vi "Vision Processing.vi"(4 "error in (no error)":errorcluster, 6 "CameraDevRef":T1) -> ()   [LabVIEW 2011]
uses:
  <vilib>/Rock Robotics/WPI/Camera/WPI_CameraDevRef.ctl
  Robot Global Data.vi
  <vilib>/vision/NI_Vision_Development_Module.lvlib
panel:
  in  "Y AbsolVal Difference":dbl=0.25
  in  "Default Shooter Speed Dump":dbl=0.42
  in  "Default Shooter Speed Shoot":dbl=1.0
  in  "Scale":dbl=0.85
  in  "Minimum Power":dbl=0.22
  out "Aspect Ratio":dbl[](array[numeric])
  out "Offset":dbl
  out "Raw Turret":dbl
  out "Target X Coord":dbl
  out "Target Distance":dbl
  out "Distance Array":dbl[](array[numeric])
  in  "Dead Band":dbl=0.09
  out "Number of Rectangles Visible":dbl
  out "Y Position Array":dbl[](array[numeric])
  out "X Position Array":dbl[](array[numeric])
  in  "View":bool
  out "Target Info":T2(array[cluster])
  in  "Area Size Limit":i32=444
  in  "Particle Count Limit":i32=8
  in  "Score Limits":T3={"Rect Coverage"=76.0, "Aspect Ratio"=40.0, "X Edge Strength"=40.0, "Y Edge Strength"=60.0}
  in  "Processing":enum32{"Color", "Intensity", "Intensity Open"}(tab)=enum."Intensity"
  in  "Luminance":i32=255
  in  "Saturation":i32=255
  in  "Hue":i32(knob)=65 scale=0.0..255.0
  in  "Margins":cluster{"Hue":i32, "Sat":i32, "Lum":i32}={"Hue"=20, "Sat"=27, "Lum"=30} {"Sat" scale=0.0..40.0; "Lum" scale=0.0..40.0; "Hue" scale=0.0..40.0}
  in  "Range":cluster{"Lower value":sgl, "Upper value":sgl}={"Lower value"=151.52174, "Upper value"=255.0} {"Lower value" scale=0.0..255.0; "Upper value" scale=0.0..255.0}
  in  "Range":cluster{"Lower value":sgl, "Upper value":sgl}={"Lower value"=123.804344, "Upper value"=255.0} {"Lower value" scale=0.0..255.0; "Upper value" scale=0.0..255.0}
  in  "View":bool
  out "Processed Image":T4(plugin-control)
  out "Original Image":T4(plugin-control)
  # "Instructions:\nProcessing the reflective tape that is illuminated by a ring light can be based\non color or light intensity.\nParticles within the image are scored by rectangle coverage, aspect ratio, and\nfor being hollow with a bold edge. A particle is considered a target if all scores\nare above the score limits. Particles can be annotated -- surrounded by\na rectangle and scores drawn to the left .\nTo control the number of particles being scored, use the count limit and the size\nlimit."
  # "(in)"
  # "To debug, Enable using the View button.\nFor color processing, you can click in the image to select the color for processing."
  # "Enable by clicking the View button.\nGreen scores are above the limit, orange are below. Inner/outer rect\nindicates all passed."
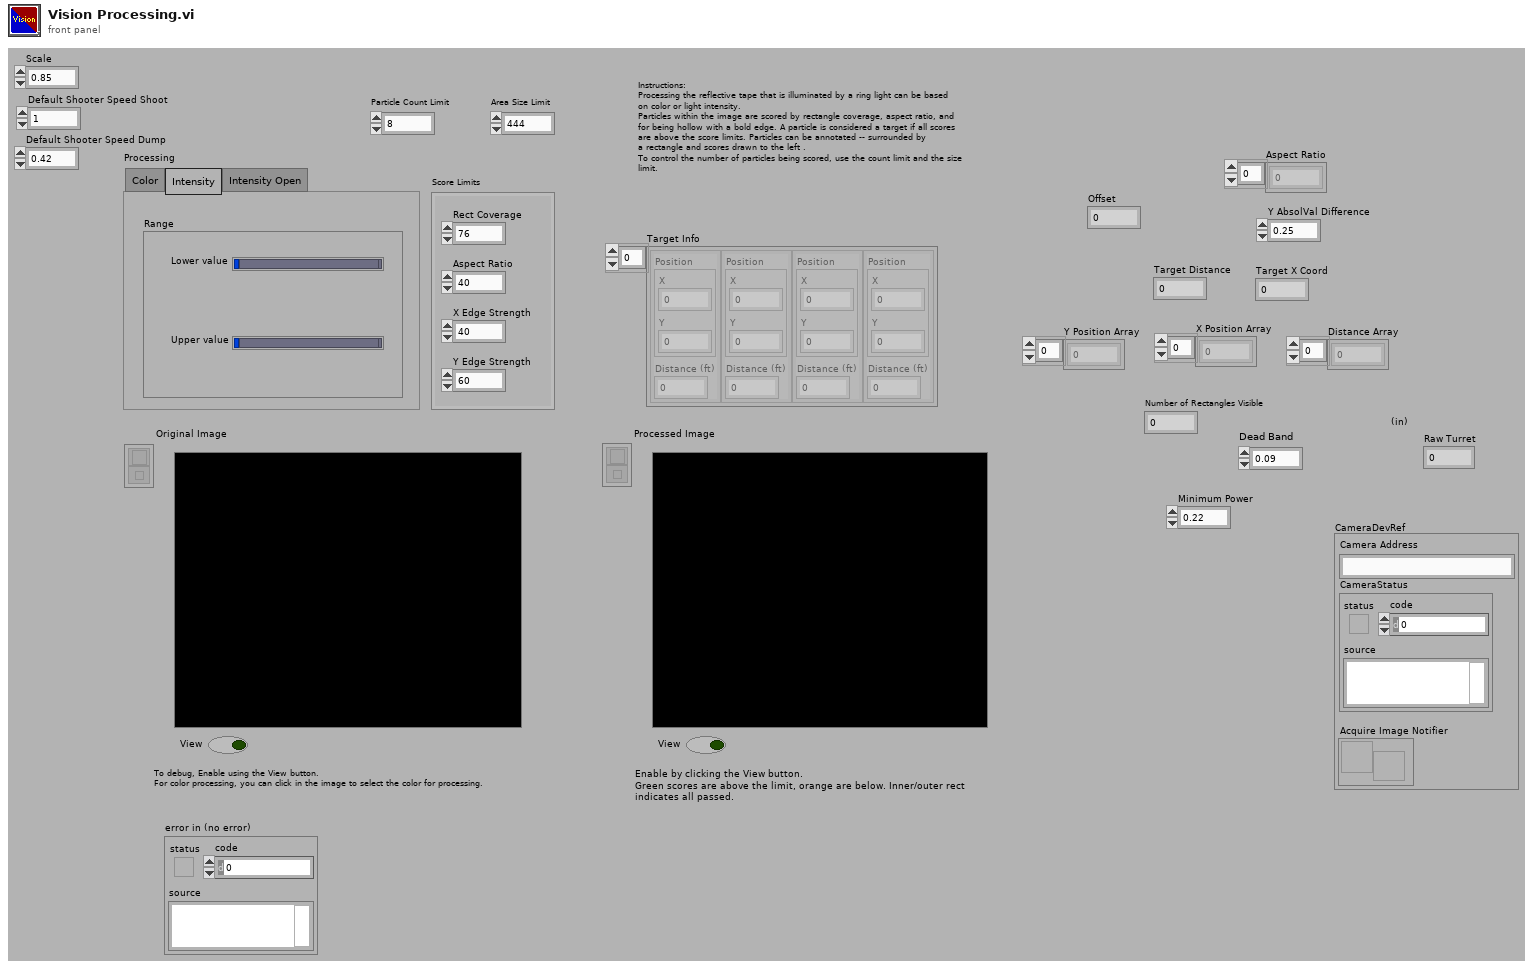
[diagram p1: front panel]
types:
  T1 = typedef "WPI_CameraDevRef.ctl" = cluster{"Camera Address":string, "CameraStatus":errorcluster, "Acquire Image Notifier":refnum<notifier>}
  T2 = cluster{"Position":cluster{"X":dbl, "Y":dbl}, "Distance (ft)":dbl}[]
  T3 = cluster{"Rect Coverage":dbl, "Aspect Ratio":dbl, "X Edge Strength":dbl, "Y Edge Strength":dbl}
  T4 = typedef "IMAQ Image.ctl" = refnum<image>
  T5 = typedef "Image Type" = u32
  T6 = enum32{"AutoM", "Close", "Dilate", "Erode", "Gradient", "Gradient out", "Gradient in", "Hit miss", "Open", "PClose", "POpen", "Thick", "Thin"}
  T7 = typedef "WPI_CameraImageSize.ctl" = enum16{"640x480", "320x240", "160x120"}
  T8 = cluster{"fps":i32, "compression":i32, "Image Size":T7}
  T9 = cluster{cluster{"Left":dbl, "Top":dbl, "Right":dbl, "Bottom":dbl}, dbl[]}[]
  T10 = cluster{"Left":dbl, "Top":dbl, "Right":dbl, "Bottom":dbl}
  T11 = cluster{"Target Center (-1 to 1)":cluster{"X":dbl, "Y":dbl}, "Distance (ft)":dbl}
  T12 = cluster{"Target Center (-1 to 1)":cluster{"X":dbl, "Y":dbl}, "Distance (ft)":dbl}[]
  T13 = typedef "WPI_JoystickDevRef.ctl" = cluster{"Device":T14}
  T14 = typedef "WPI_JoystickDeviceEnum.ctl" = enum16{"USB 1", "USB 2", "USB 3", "USB 4", "Kinect 1", "Kinect 2"}
  T15 = typedef "WPI_JoystickButtonState.ctl" = cluster{"Button 1":bool, "Button 2":bool, "Button 3":bool, "Button 4":bool, "Button 5":bool, "Button 6":bool, "Button 7":bool, "Button 8":bool, "Button 9":bool, "Button 10":bool, "Button 11":bool, "Button 12":bool}
  T16 = cluster{"axis 1 (x)":dbl, "axis 2 (y)":dbl, "axis 3 (throttle)":dbl, "axis 4":dbl, "axis 5":dbl, "axis 6":dbl}
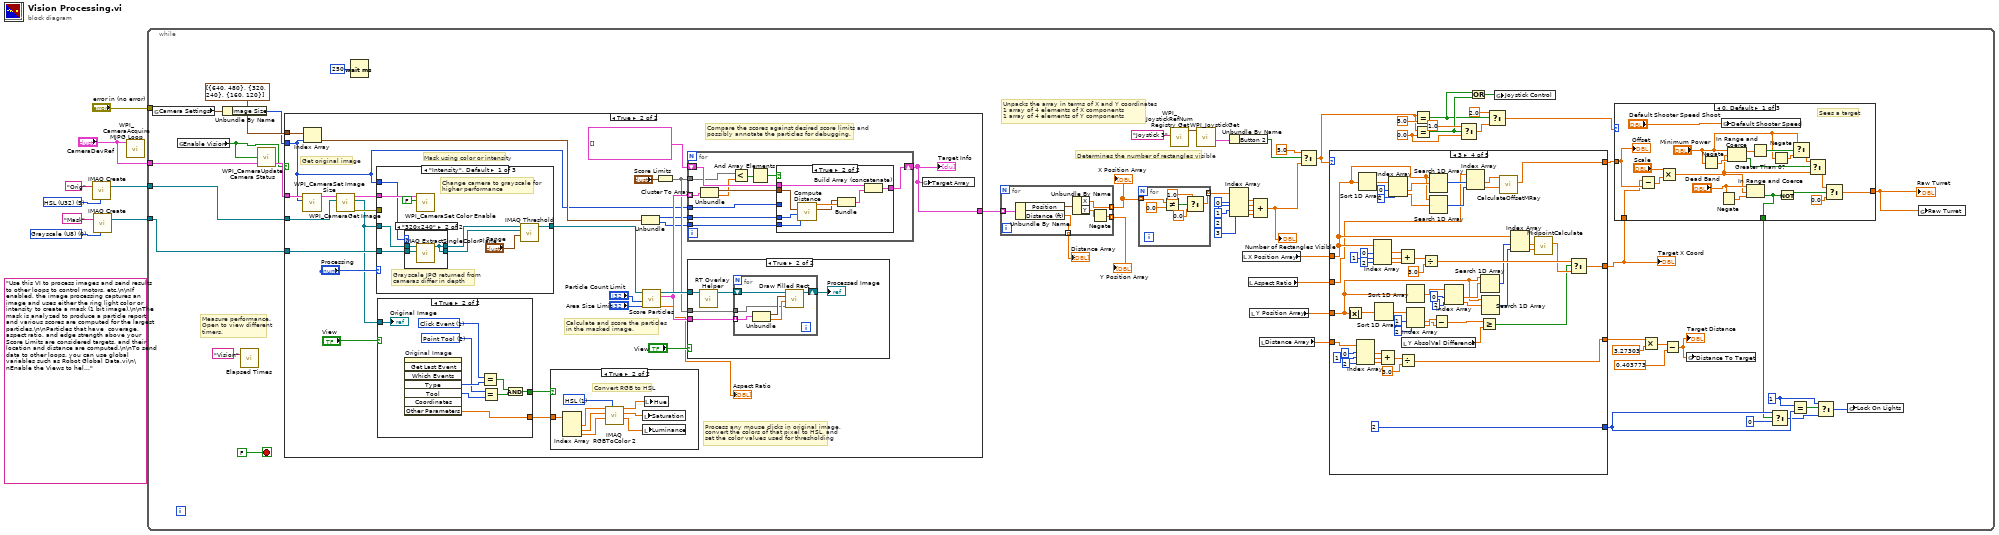
[diagram p0: block diagram]
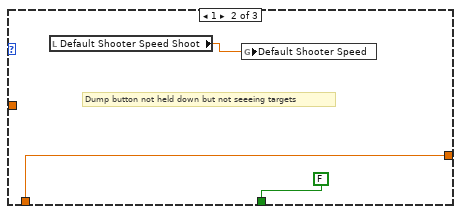
[diagram p2: hidden frame]
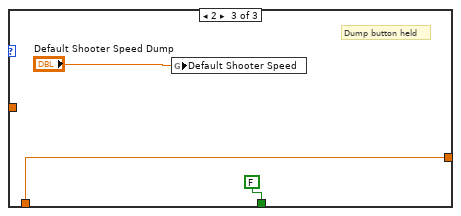
[diagram p3: hidden frame]
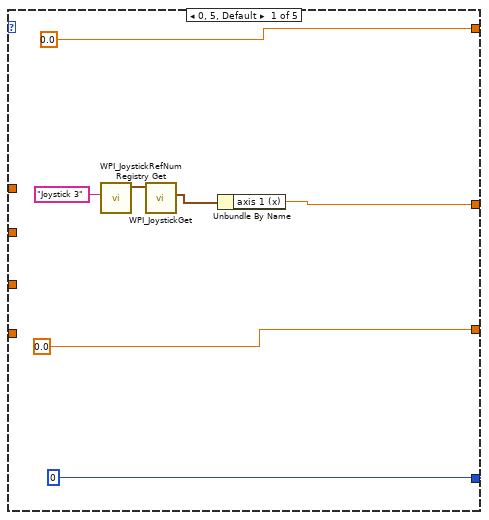
[diagram p4: hidden frame]
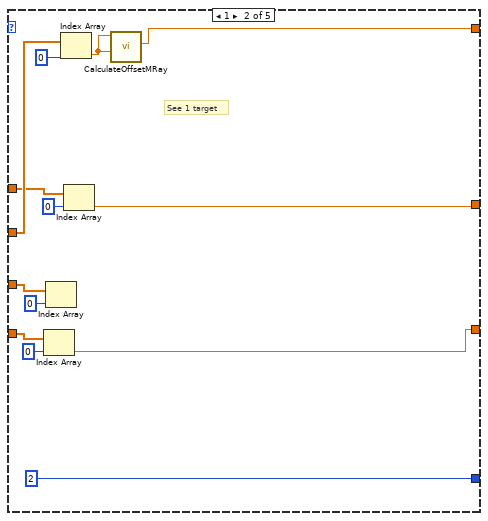
[diagram p5: hidden frame]
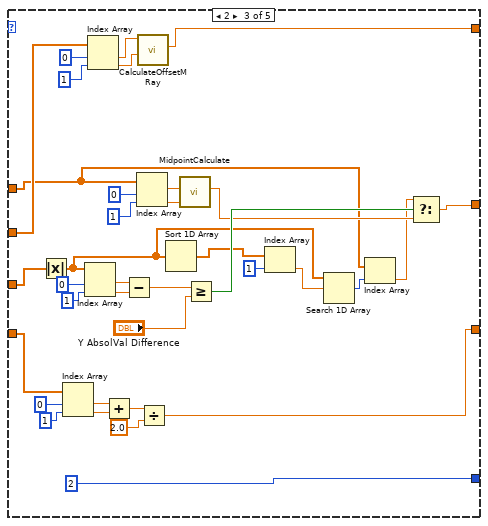
[diagram p6: hidden frame]
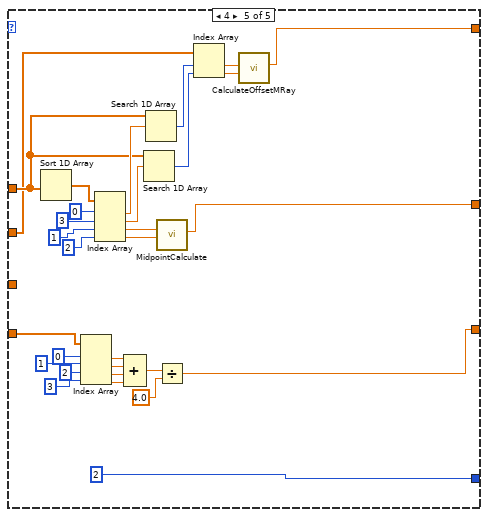
[diagram p7: hidden frame]
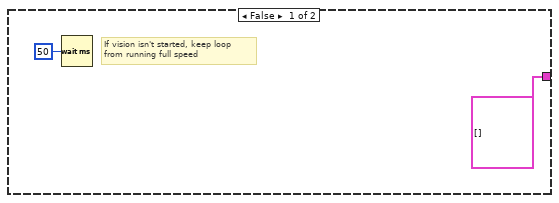
[diagram p8: hidden frame]
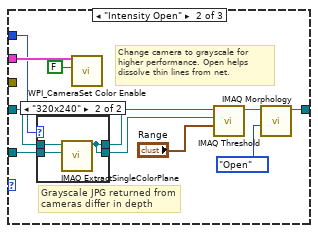
[diagram p11: hidden frame]
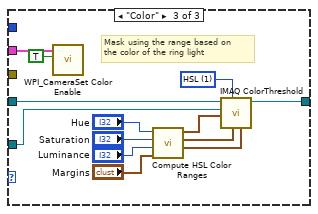
[diagram p13: hidden frame]
diagram:
  w3 = T5 0 items=["Grayscale (U8)", "Grayscale (I16)", "Grayscale (SGL)", "Complex (CSG)", "RGB (U32)", "HSL (U32)", "RGB (U64)", "Grayscale (U16)"] ("Image Type")
  (unwired) "Use this VI to process images and send results to other loops to control motors, etc.\n\nIf enabled, the image processing captures an image and uses either the ring light color or intensity to create a mask (1 bit image).\n\nThe mask is analyzed to produce a particle report and various scores are computed for the largest particles.\n\nParticles that have  coverage, aspect ratio, and edge strength above your Score Limits are considered targets, and their location and distance are computed.\n\nTo send data to other loops, you can use global variables such as Robot Global Data.vi\n\nEnable the Views to help debug color settings. Disable the View to speed up processing."
  w7 = T5 5 items=["Grayscale (U8)", "Grayscale (I16)", "Grayscale (SGL)", "Complex (CSG)", "RGB (U32)", "HSL (U32)", "RGB (U64)", "Grayscale (U16)"] ("Image Type")
  n1 = call "IMAQ Create"("Image Name"="Orig", "Image Type"=w7) -> ("New Image"=w6:T4)  [unwired: 2 in, 2 out]
  n2 = call "IMAQ Create"("Image Name"="Mask", "Image Type"=w3) -> ("New Image"=w1:T4)  [unwired: 2 in, 2 out]
  n3 = call <vilib>:"WPI_CameraAcquire MJPG Loop.vi"("CameraDevRef"="CameraDevRef") -> ()  [unwired: 11 in]
  n4 = while {
    tunnel: w6 -> [w66]
    tunnel: "CameraDevRef" -> [w65]
    tunnel: "error in (no error)" -> [_]
    tunnel: w1 -> [w61]
    stop <- FALSE stop-if-true
    w14 = 0.0 ("y")
    w31 = 1 ("y")
    # "Determines the number of rectangles visible"
    # "Unpacks the array in terms of X and Y coordinates\n1 array of 4 elements of X components\n1 array of 4 elements of Y components"
    # "Measure performance.\nOpen to view different\ntimers."
    n5 = global read "Robot Global Data.vi" "Camera Settings"() -> (w59:T8)
    n6 = global read "Robot Global Data.vi" "Enable Vision"() -> (w63:bool)
    n7 = Unbundle By Name(w59) -> ("Image Size"=w58:T7)
    n8 = call "Elapsed Times.vi"("Call Name"="Vision") -> ()  [unwired: 2 in, 1 out]
    n9 = call <vilib>:"WPI_CameraUpdate Camera Status.vi"("CameraDevRef In"=w65, "Enable Vision"=w63) -> ("CameraDevRef Out"=w64:T1)  [unwired: 3 in]
    n10 = case shown="True" w63 {
      tunnel: w66 -> [_ w264]
      tunnel: w64 -> [_ w260]
      tunnel: w61 -> [_ w251]
      tunnel: cluster{i32, i32}[] [{640, 480}, {320, 240}, {160, 120}] -> [_ w255]
      tunnel: w58 -> [_ w248]
      tunnel: [T2 [] w249] -> w57
      frame False {
        # "If vision isn't started, keep loop\nfrom running full speed"
        n11 = Wait (ms)(milliseconds to wait=u32 50) -> ()  [unwired: 1 out]
      }
      frame True {
        # "Compare the scores against desired score limits and\npossibly annotate the particles for debugging."
        # "Process any mouse clicks in original image,\nconvert the colors of that pixel to HSL, and\nset the color values used for thresholding"
        # "Calculate and score the particles\nin the masked image."
        # "Mask using color or intensity"
        # "Get original image"
        n12 = call <vilib>:"WPI_CameraSet Image Size.vi"("Image Size"=w248, "CameraDevRef"=w260) -> ("CameraDevRef Out"=w261:T1)  [unwired: 8 in, 1 out]
        n13 = Index Array(array=w255, index=w248) -> (element=w252:cluster{i32, i32})
        n14 = call <vilib>:"WPI_CameraGet Image.vi"("Image"=w264, "CameraDevRef"=w261) -> ("error out"=w262:errorcluster, "Image Out"=w250:T4, "CameraDevRef Out"=w263:T1)  [unwired: 7 in]
        n15 = case shown="\"Intensity\", Default" "Processing" {
          tunnel: w250 -> [w286 w298 w324]
          tunnel: [w289 w303 w323] -> w258
          tunnel: w263 -> [w287 w301 w314]
          tunnel: w262 -> [_ _ _]
          tunnel: w251 -> [w285 w299 w312]
          tunnel: w248 -> [w284 w300 _]
          frame "Intensity", Default {
            # "Grayscale JPG returned from\ncameras differ in depth"
            # "Change camera to grayscale for\nhigher performance"
            n16 = case shown="\"320x240\"" w284 {
              tunnel: w286 -> [w292 w295]
              tunnel: w285 -> [w291 w294]
              tunnel: [w292 w293] -> w283
              tunnel: [w291 w293] -> w282
              frame "640x480", Default {
              }
              frame "320x240" {
                n17 = call "IMAQ ExtractSingleColorPlane"("Image Dst"=w294, "Image Src"=w295) -> ("Image Dst Out"=w293:T4)  [unwired: 8 in, 1 out]
              }
            }
            n18 = call <vilib>:"WPI_CameraSet Color Enable.vi"("Color Enabled"=FALSE, "CameraDevRef"=w287) -> ()  [unwired: 8 in, 2 out]
            n19 = call "IMAQ Threshold"("Range"="Range", "Image Dst"=w282, "Image Src"=w283) -> ("Image Dst Out"=w289:T4)  [unwired: 3 in, 5 out]
          }
          frame "Intensity Open" {
            # "Grayscale JPG returned from\ncameras differ in depth"
            # "Change camera to grayscale for\nhigher performance. Open helps\ndissolve thin lines from net."
            n20 = case shown="\"320x240\"" w300 {
              tunnel: w298 -> [w308 w311]
              tunnel: w299 -> [w307 w310]
              tunnel: [w308 w309] -> w297
              tunnel: [w307 w309] -> w296
              frame "640x480", Default {
              }
              frame "320x240" {
                n21 = call "IMAQ ExtractSingleColorPlane"("Image Dst"=w310, "Image Src"=w311) -> ("Image Dst Out"=w309:T4)  [unwired: 8 in, 1 out]
              }
            }
            n22 = call <vilib>:"WPI_CameraSet Color Enable.vi"("Color Enabled"=FALSE, "CameraDevRef"=w301) -> ()  [unwired: 8 in, 2 out]
            n23 = call "IMAQ Threshold"("Range"="Range", "Image Dst"=w296, "Image Src"=w297) -> ("Image Dst Out"=w304:T4)  [unwired: 3 in, 5 out]
            n24 = call "IMAQ Morphology"("Operation"=T6."Open", "Image Src"=w304) -> ("Image Dst Out"=w303:T4)  [unwired: 8 in, 1 out]
          }
          frame "Color" {
            w322 = u16 1 items=["RGB", "HSL", "HSV", "HSI"] ("Color Mode")
            # "Mask using the range based on\nthe color of the ring light"
            n25 = call <vilib>:"WPI_CameraSet Color Enable.vi"("Color Enabled"=TRUE, "CameraDevRef"=w314) -> ()  [unwired: 8 in, 2 out]
            n26 = call "Compute HSL Color Ranges.vi"("Margins"="Margins", "Luminance"="Luminance", "Saturation"="Saturation", "Hue"="Hue") -> ("Lum Range"=w319:cluster{i32, i32}, "Sat Range"=w320:cluster{i32, i32}, "Hue Range"=w321:cluster{i32, i32})  [unwired: 5 in]
            n27 = call "IMAQ ColorThreshold"("Blue or Luma or Val or Inten Range"=w319, "Green or Sat Range"=w320, "Color Mode"=w322, "Red or Hue Range"=w321, "Image Dst"=w312, "Image Src"=w324) -> ("Image Dst Out"=w323:T4)  [unwired: 4 in, 1 out]
          }
        }
        n28 = case shown="True" "View" {
          tunnel: w250 -> [_ w344]
          tunnel: [_ w339] -> w257
          tunnel: [_ w336] -> w256
          frame False {
          }
          frame True {
            w337 = 2 items=["None", "Selection Tool", "Point Tool", "Line Tool", "Rectangle Tool", "Oval Tool", "Polygon Tool", "ClosedFreehandTool", "Annulus Tool", "Rotated Rectangle Tool", "Zoom Tool", "Pan Tool", "Polyline Tool", "Freehand Tool"] ("Tool")
            w338 = 1 items=["No Event"=0, "Click Event"=1, "Draw Event"=2, "Size Event"=4, "Scroll Event"=5, "Double Click Event"=8] ("Type")
            n29 = invoke on="Original Image" class="ImageControl" method="Get Last Event"() -> ("Type"=w340:i32, "Tool"=w343:i32, "Other Parameters"=w336:sgl[])  [unwired: 8 in, 5 out]
            n30 = Equal?(x=w338, y=w340) -> (x = y?=w341:bool)
            n31 = Equal?(x=w337, y=w343) -> (x = y?=w342:bool)
            n32 = And(x=w341, y=w342) -> (x .and. y?=w339:bool)
            "Original Image" <- w344
          }
        }
        n33 = case shown="True" w257 {
          tunnel: w256 -> [_ w281]
          frame False {
          }
          frame True {
            w280 = u16 1 items=["RGB", "HSL", "HSV", "HSI", "CIE L*a*b*", "CIE XYZ"] ("Color Mode")
            # "Convert RGB to HSL"
            n34 = Index Array(array=w281) -> (element #1=w279:sgl, element #2=w277:sgl, element #3=w275:sgl)  [unwired: 3 in]
            n35 = call "IMAQ RGBToColor 2"("Color Mode"=w280, "Blue value"=w275, "Green value"=w277, "Red value"=w279) -> ("Blue or Luma or Val or Inten or Z or b*value"=w274:dbl, "Green or Sat or Y or a* value"=w276:dbl, "Red or Hue or X or L* value"=w278:dbl)  [unwired: 4 in, 1 out]
            n36 = local write "Saturation"(w276) -> ()
            n37 = local write "Luminance"(w274) -> ()
            n38 = local write "Hue"(w278) -> ()
          }
        }
        n39 = Unbundle(w252) -> (w254:i32, w253:i32)
        n40 = call "Score Particles.vi"("Area Size Limit"="Area Size Limit", "Particle Count Limit"="Particle Count Limit", "Image Refnum in"=w258) -> ("Aspect Ratio"=→"Aspect Ratio":dbl[], "Scored Particle Info"=w269:T9, "Image Refnum out"=w272:T4)  [unwired: 6 in]
        n41 = Cluster To Array(cluster="Score Limits") -> (array=w267:dbl[])
        n42 = for {
          shift-right: [w354] -> w249
          shift-left: T2 [] -> [w355]
          tunnel: w254 -> [w353]
          tunnel: w269 -> [w351] mode=indexing
          tunnel: w267 -> [w346]
          tunnel: w248 -> [w350]
          tunnel: w253 -> [w345]
          n43 = Unbundle(w351) -> (w352:T10, w347:dbl[])
          n44 = Less?(x=w346, y=w347) -> (x < y?=w349:bool[])
          n45 = And Array Elements(Boolean array=w349) -> (logical AND=w348:bool)
          n46 = case shown="True" w348 {
            tunnel: w355 -> [w356 w364]
            tunnel: [w356 w363] -> w354
            tunnel: w352 -> [_ w359]
            tunnel: w353 -> [_ w361]
            tunnel: w350 -> [_ _]
            tunnel: w345 -> [_ w358]
            frame False {
            }
            frame True {
              n47 = call "Compute Distance.vi"("Y Image Resolution"=w358, "X Image Resolution"=w361, "Bounding Box"=w359) -> ("Target Center (-1 to 1)"=w357:cluster{"X":dbl, "Y":dbl}, "Distance (ft)"=w360:dbl)  [unwired: 7 in]
              n48 = Bundle("Target Center (-1 to 1)"=w357, "Distance (ft)"=w360) -> (w362:T11)  [unwired: 1 in]
              n49 = Build Array (concatenate)(w364, w362) -> (w363:T12)
            }
          }
        }
        "Target Info" <- w249
        n50 = case shown="True" "View" {
          tunnel: w272 -> [_ w326]
          tunnel: w269 -> [_ w328]
          tunnel: w267 -> [_ w327]
          frame False {
          }
          frame True {
            n51 = call "RT Overlay Helper.vi"("Refnum in"=w326) -> ("Refnum out"=w329:T4)  [unwired: 10 in]
            n52 = for {
              shift-right: [w334] -> w325
              shift-left: w329 -> [w335]
              tunnel: w328 -> [w331] mode=indexing
              tunnel: w327 -> [w330]
              n53 = Unbundle(w331) -> (w332:T10, w333:dbl[])
              n54 = call "Draw Filled Rect.vi"("Limits"=w330, "Scores"=w333, "Bounding Box"=w332, "image in"=w335) -> ("image out"=w334:T4)  [unwired: 7 in]
            }
            "Processed Image" <- w325
          }
        }
        n55 = global write "Robot Global Data.vi" "Target Array"(w249) -> ()
      }
    }
    n56 = Wait (ms)(milliseconds to wait=u32 250) -> ()  [unwired: 1 out]
    n57 = for {
      tunnel: [w242] -> w37 mode=indexing
      tunnel: [w243] -> w47 mode=indexing
      tunnel: w57 -> [w240] mode=indexing
      tunnel: [w239] -> w49 mode=indexing
      n58 = Unbundle By Name(w240) -> ("Position"=w244:cluster{"X":dbl, "Y":dbl}, "Distance (ft)"=w239:dbl)
      n59 = Unbundle By Name(w244) -> ("X"=w243:dbl, "Y"=w241:dbl)
      n60 = Negate(x=w241) -> (-x=w242:dbl)
    }
    "X Position Array" <- w47
    "Y Position Array" <- w37
    "Distance Array" <- w49
    n61 = for {
      tunnel: w47 -> [w98] mode=indexing
      tunnel: [w94] -> w46 mode=indexing
      n62 = Not Equal?(x=w98, y=0.0) -> (x != y?=w97:bool)
      n63 = Select(t=1.0, s=w97, f=0.0) -> (s? t:f=w94:dbl)
    }
    n64 = call <vilib>:"WPI_JoystickRefNum Registry Get.vi"("refnum name"="Joystick 3") -> ("JoystickDevRef"=w36:T13)  [unwired: 9 in, 1 out]
    n65 = call <vilib>:"WPI_JoystickGet.vi"("JoystickDevRef"=w36) -> ("Buttons"=w34:T15)  [unwired: 4 in, 2 out]
    n66 = Unbundle By Name(w34) -> ("Button 2"=w33:bool)
    n67 = Index Array(array=w46, index #1=0 ("index"), index #2=1 ("index"), index #3=2 ("index"), index #4=3 ("index")) -> (element #1=w44:dbl, element #2=w45:dbl, element #3=w43:dbl, element #4=w42:dbl)
    n68 = local read "X Position Array"() -> (w48:dbl[])
    n69 = local read "Aspect Ratio"() -> (w26:dbl[])
    n70 = local read "Y Position Array"() -> (w50:dbl[])
    n71 = Compound Arithmetic op=ADD(w44, w45, w43, w42) -> (w27:dbl)
    "Number of Rectangles Visible" <- w27
    n72 = local read "Distance Array"() -> (w51:dbl[])
    n73 = Select(t=5.0, s=w33, f=w27) -> (s? t:f=w13:dbl)
    n74 = case shown="3" w13 {
      tunnel: w48 -> [_ w114 w121 w163 w214]
      tunnel: [w102 w113 w145 w197 w237] -> w24
      tunnel: w50 -> [_ w111 w144 w175 _]
      tunnel: w51 -> [_ w109 w133 w206 w234]
      tunnel: [0 2 2 2 2] -> w30
      tunnel: [0.0 ("Offset") w116 w150 w156 w223] -> w25
      tunnel: w26 -> [_ w119 w153 w159 w209]
      tunnel: [0.0 w108 w128 w199 w224] -> w19
      frame 0, 5, Default {
        n75 = call <vilib>:"WPI_JoystickRefNum Registry Get.vi"("refnum name"="Joystick 3") -> ("JoystickDevRef"=w101:T13)  [unwired: 9 in, 1 out]
        n76 = call <vilib>:"WPI_JoystickGet.vi"("JoystickDevRef"=w101) -> ("Axes"=w103:T16)  [unwired: 4 in, 2 out]
        n77 = Unbundle By Name(w103) -> ("axis 1 (x)"=w102:dbl)
      }
      frame 1 {
        # "See 1 target"
        n78 = Index Array(array=w109, index=0) -> (element=w108:dbl)
        n79 = Index Array(array=w111, index=0) -> ()  [unwired: 1 out]
        n80 = Index Array(array=w119, index=0) -> (element=w117:dbl)
        n81 = Index Array(array=w114, index=0) -> (element=w113:dbl)
        n82 = call "CalculateOffsetMRay.vi"("AR2"=w117, "AR1"=w117) -> ("Offset"=w116:dbl)  [unwired: 9 in]
      }
      frame 2 {
        n83 = Absolute Value(x=w144) -> (abs(x)=w124:dbl[])
        n84 = Index Array(array=w133, index #1=0 ("index"), index #2=1 ("index")) -> (element #1=w131:dbl, element #2=w132:dbl)
        n85 = Index Array(array=w124, index #1=0 ("index"), index #2=1 ("index")) -> (element #1=w140:dbl, element #2=w141:dbl)
        n86 = Index Array(array=w153, index #1=0 ("index"), index #2=1 ("index")) -> (element #1=w152:dbl, element #2=w151:dbl)
        n87 = Add(x=w131, y=w132) -> (x+y=w130:dbl)
        n88 = Subtract(x=w140, y=w141) -> (x-y=w139:dbl)
        n89 = Index Array(array=w121, index #1=0 ("index"), index #2=1 ("index")) -> (element #1=w146:dbl, element #2=w147:dbl)
        n90 = call "CalculateOffsetMRay.vi"("AR2"=w151, "AR1"=w152) -> ("Offset"=w150:dbl)  [unwired: 9 in]
        n91 = Divide(x=w130, y=2.0) -> (x/y=w128:dbl)
        n92 = Sort 1D Array(array=w124) -> (sorted array=w126:dbl[])
        n93 = call "MidpointCalculate.vi"("X2"=w147, "X1"=w146) -> ("Midpoint"=w136:dbl)  [unwired: 9 in]
        n94 = Greater Or Equal?(x=w139, y="Y AbsolVal Difference") -> (x >= y?=w137:bool)
        n95 = Index Array(array=w126, index=1) -> (element=w123:dbl)
        n96 = Search 1D Array(1D array=w124, element=w123) -> (index of element=w122:i32)  [unwired: 1 in]
        n97 = Index Array(array=w121, index=w122) -> (element=w120:dbl)
        n98 = Select(t=w120, s=w137, f=w136) -> (s? t:f=w145:dbl)
      }
      frame 3 {
        n99 = Absolute Value(x=w175) -> (abs(x)=w196:dbl[])
        n100 = Index Array(array=w206, index #1=0 ("index"), index #2=1 ("index"), index #3=2 ("index")) -> (element #1=w202:dbl, element #2=w203:dbl, element #3=w204:dbl)
        n101 = Sort 1D Array(array=w163) -> (sorted array=w167:dbl[])
        n102 = Index Array(array=w163, index #1=0 ("index"), index #2=1 ("index"), index #3=2 ("index")) -> (element #1=w184:dbl, element #2=w186:dbl, element #3=w185:dbl)
        n103 = Sort 1D Array(array=w196) -> (sorted array=w180:dbl[])
        n104 = Compound Arithmetic op=ADD(w202, w203, w204) -> (w201:dbl)
        n105 = Index Array(array=w167, index #1=0 ("index"), index #2=2 ("index")) -> (element #1=w164:dbl, element #2=w162:dbl)
        n106 = Divide(x=w201, y=3.0) -> (x/y=w199:dbl)
        n107 = Compound Arithmetic op=ADD(w184, w186, w185) -> (w183:dbl)
        n108 = local read "Y AbsolVal Difference"() -> (w190:dbl)
        n109 = Sort 1D Array(array=w175) -> (sorted array=w179:dbl[])
        n110 = Index Array(array=w180, index #1=1 ("index"), index #2=2 ("index")) -> (element #1=w192:dbl, element #2=w193:dbl)
        n111 = Divide(x=w183, y=3.0) -> (x/y=w181:dbl)
        n112 = Search 1D Array(1D array=w163, element=w164) -> (index of element=w161:i32)  [unwired: 1 in]
        n113 = Search 1D Array(1D array=w163, element=w162) -> (index of element=w160:i32)  [unwired: 1 in]
        n114 = Subtract(x=w193, y=w192) -> (x-y=w191:dbl)
        n115 = Index Array(array=w179, index #1=0 ("index"), index #2=2 ("index")) -> (element #1=w176:dbl, element #2=w174:dbl)
        n116 = Index Array(array=w159, index #1=w161, index #2=w160) -> (element #1=w158:dbl, element #2=w157:dbl)
        n117 = Greater Or Equal?(x=w191, y=w190) -> (x >= y?=w168:bool)
        n118 = Search 1D Array(1D array=w175, element=w176) -> (index of element=w173:i32)  [unwired: 1 in]
        n119 = Search 1D Array(1D array=w175, element=w174) -> (index of element=w172:i32)  [unwired: 1 in]
        n120 = call "CalculateOffsetMRay.vi"("AR2"=w157, "AR1"=w158) -> ("Offset"=w156:dbl)  [unwired: 9 in]
        n121 = Index Array(array=w163, index #1=w173, index #2=w172) -> (element #1=w170:dbl, element #2=w171:dbl)
        n122 = call "MidpointCalculate.vi"("X2"=w171, "X1"=w170) -> ("Midpoint"=w169:dbl)  [unwired: 9 in]
        n123 = Select(t=w181, s=w168, f=w169) -> (s? t:f=w197:dbl)
      }
      frame 4 {
        n124 = Sort 1D Array(array=w214) -> (sorted array=w238:dbl[])
        n125 = Index Array(array=w234, index #1=0 ("index"), index #2=1 ("index"), index #3=2 ("index"), index #4=3 ("index")) -> (element #1=w231:dbl, element #2=w230:dbl, element #3=w229:dbl, element #4=w228:dbl)
        n126 = Index Array(array=w238, index #1=0 ("index"), index #2=3 ("index"), index #3=1 ("index"), index #4=2 ("index")) -> (element #1=w215:dbl, element #2=w216:dbl, element #3=w222:dbl, element #4=w221:dbl)
        n127 = Compound Arithmetic op=ADD(w231, w230, w229, w228) -> (w227:dbl)
        n128 = Search 1D Array(1D array=w214, element=w216) -> (index of element=w211:i32)  [unwired: 1 in]
        n129 = Search 1D Array(1D array=w214, element=w215) -> (index of element=w210:i32)  [unwired: 1 in]
        n130 = call "MidpointCalculate.vi"("X2"=w221, "X1"=w222) -> ("Midpoint"=w237:dbl)  [unwired: 9 in]
        n131 = Divide(x=w227, y=4.0) -> (x/y=w224:dbl)
        n132 = Index Array(array=w209, index #1=w210, index #2=w211) -> (element #1=w213:dbl, element #2=w212:dbl)
        n133 = call "CalculateOffsetMRay.vi"("AR2"=w212, "AR1"=w213) -> ("Offset"=w223:dbl)  [unwired: 9 in]
      }
    }
    "Target X Coord" <- w24
    n134 = Equal?(x=w13, y=5.0) -> (x = y?=w11:bool)
    n135 = Equal?(x=w13, y=w14) -> (x = y?=w12:bool)
    n136 = Select(t=1.0, s=w12, f=w14) -> (s? t:f=w17:dbl)
    n137 = Or(x=w11, y=w12) -> (x .or. y?=w10:bool)
    n138 = Select(t=2.0, s=w11, f=w17) -> (s? t:f=w9:dbl)
    n139 = global write "Robot Global Data.vi" "Joystick Control"(w10) -> ()
    n140 = case shown="0, Default" w9 {
      tunnel: w25 -> [w86 _ _]
      tunnel: w24 -> [w85 w90 w93]
      tunnel: [w68 w90 w93] -> w55
      tunnel: [w71 FALSE FALSE] -> w23
      frame 0, Default {
        # "Sees a target"
        n141 = Subtract(x=w85, y=w86) -> (x-y=w83:dbl)
        n142 = Multiply(x="Scale", y=w83) -> (x*y=w74:dbl)
        n143 = Negate(x="Minimum Power") -> (-x=w81:dbl)
        n144 = Negate(x="Dead Band") -> (-x=w87:dbl)
        n145 = global write "Robot Global Data.vi" "Default Shooter Speed"("Default Shooter Speed Shoot") -> ()
        n146 = In Range and Coerce(upper limit="Minimum Power", x=w74, lower limit=w81) -> (coerced(x)=w77:dbl, In Range?=w78:bool)
        n147 = In Range and Coerce(upper limit="Dead Band", x=w74, lower limit=w87) -> (In Range?=w71:bool)  [unwired: 1 out]
        n148 = Greater Than 0?(x=w77) -> (x > 0?=w76:bool)
        n149 = Negate(x="Minimum Power") -> (-x=w73:dbl)
        n150 = Not(x=w71) -> (.not. x?=w72:bool)
        n151 = Select(t="Minimum Power", s=w76, f=w73) -> (s? t:f=w75:dbl)
        n152 = Select(t=w75, s=w78, f=w74) -> (s? t:f=w79:dbl)
        n153 = Select(t=w79, s=w72, f=0.0) -> (s? t:f=w68:dbl)
        "Offset" <- w86
      }
      frame 1 {
        # "Dump button not held down but not seeeing targets"
        n154 = local read "Default Shooter Speed Shoot"() -> (w88:dbl)
        n155 = global write "Robot Global Data.vi" "Default Shooter Speed"(w88) -> ()
      }
      frame 2 {
        # "Dump button held"
        n156 = global write "Robot Global Data.vi" "Default Shooter Speed"("Default Shooter Speed Dump") -> ()
      }
    }
    "Raw Turret" <- w55
    n157 = Multiply(x=w19, y=3.27303) -> (x*y=w22:dbl)
    n158 = Subtract(x=w22, y=0.403773) -> (x-y=w53:dbl)
    "Target Distance" <- w53
    n159 = global write "Robot Global Data.vi" "Distance To Target"(w53) -> ()
    n160 = Select(t=w30, s=w23, f=0) -> (s? t:f=w28:i32)
    n161 = Equal?(x=w31, y=w30) -> (x = y?=w32:bool)
    n162 = Select(t=w31, s=w32, f=w28) -> (s? t:f=w54:i32)
    n163 = global write "Robot Global Data.vi" "Lock On Lights"(w54) -> ()
    n164 = global write "Robot Global Data.vi" "Raw Turret"(w55) -> ()
  }
